vi "rebuildPathFromStringArray.vi"(10 "stringArray":string[](array[string])) -> (2 "path":path)   [LabVIEW 2021]
panel:
  in  "replaceFragment":path
  in  "searchFragment":path
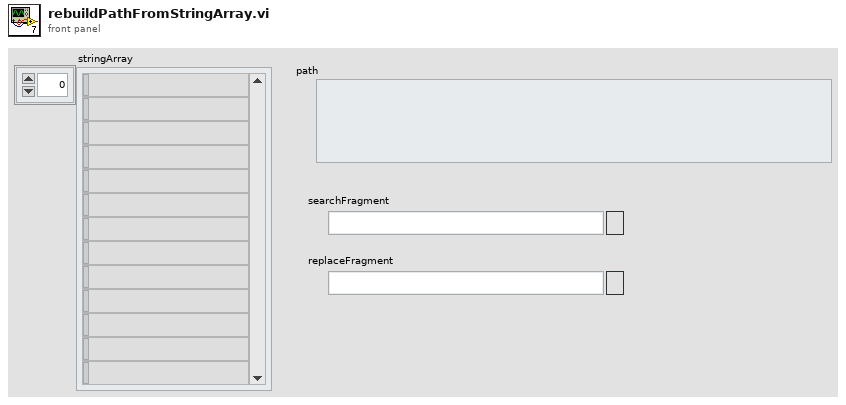
[diagram p1: front panel]
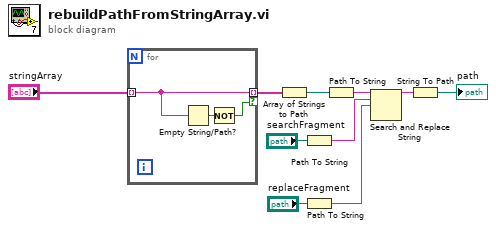
[diagram p0: block diagram]
diagram:
  n1 = for {
    tunnel: [w11] -> w10 mode=indexing if=w12
    tunnel: "stringArray" -> [w11] mode=indexing
    n2 = Empty String/Path?(string/path=w11) -> (empty?=w13:bool)
    n3 = Not(x=w13) -> (.not. x?=w12:bool)
  }
  n4 = Array of Strings to Path(0:w10) -> (2:w8:path)  [unwired: 1 in]
  n5 = Path To String(path="searchFragment") -> (string=w2:string)
  n6 = Path To String(path="replaceFragment") -> (string=w1:string)
  n7 = Path To String(path=w8) -> (string=w7:string)
  n8 = Search and Replace String(input string=w7, search string=w2, replace string=w1) -> (result string=w6:string)  [unwired: 5 in, 3 out]
  n9 = String To Path(string=w6) -> (path=→"path":path)
